vi "IRF Options.vi"() -> ()   [LabVIEW 2021, in "Fits.lvlib"]
uses:
  Fits.lvlib
panel:
  in  "Squared Multiexponential":bool
  in  "Independent Last Amplitude":bool=TRUE
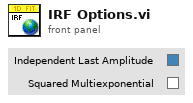
[diagram p1: front panel]
diagram:
